vi "Deadband.vi"(6 "Value":dbl, 11 "Input":dbl) -> (3 "Output":dbl)   [LabVIEW 2016]
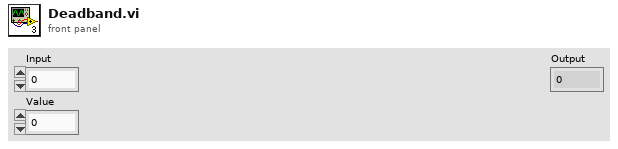
[diagram p1: front panel]
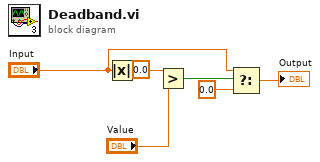
[diagram p0: block diagram]
diagram:
  (unwired) 0.0 ("x")
  n1 = Absolute Value(x="Input") -> (abs(x)=w4:dbl)
  n2 = Greater?(x=w4, y="Value") -> (0:w6:bool)
  n3 = Select(t="Input", s=w6, f=0.0) -> (s? t:f=→"Output":dbl)
